vi "test - Round Trip - Array (Empty) - Cluster.vi"(8 "error in (no error)":errorcluster, 11 "TestCase in":refnum<class "Python Data Tools Tests.lvclass">) -> (0 "error out":errorcluster, 3 "TestCase out":refnum<class "Python Data Tools Tests.lvclass">)   [LabVIEW 2013, in "Python Data Tools Tests.lvclass"]
uses:
  Python Data Tools Tests.lvclass
  <vilib>/addons/_JKI Toolkits/VI Tester/TestCase.llb/TestCase.lvclass
panel:
  out "Python String":string
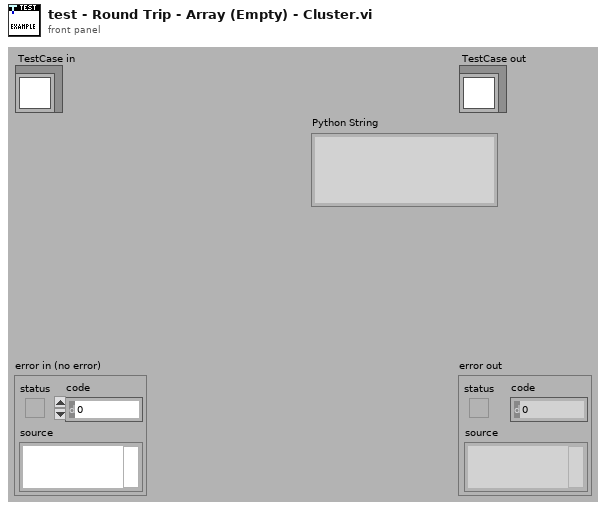
[diagram p1: front panel]
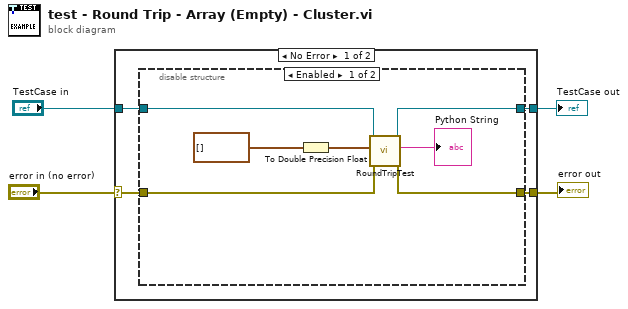
[diagram p0: block diagram]
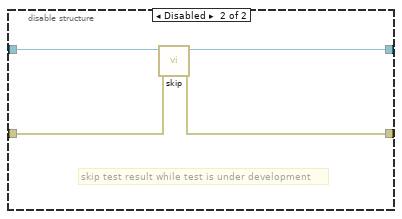
[diagram p2: hidden frame]
diagram:
  n1 = case shown="No Error" "error in (no error)" {
    selector: "error in (no error)" -> [w6 w21]
    tunnel: [w5 w21] -> w3
    tunnel: [w7 w20] -> w1
    tunnel: "TestCase in" -> [w8 w20]
    frame No Error {
      n2 = disable-structure shown="Enabled" {
        disable-tunnel: w8 -> [w15 w19]
        disable-tunnel: [w14 w16] -> w7
        disable-tunnel: w6 -> [w12 w18]
        disable-tunnel: [w13 w17] -> w5
        frame Enabled {
          n3 = To Double Precision Float(number=cluster{dbl}[] []) -> (double precision float=w11:cluster{dbl}[])
          n4 = call "RoundTripTest.vi"("error in (no error)"=w12, "Variant"=w11, "TestCase in"=w15) -> ("error out"=w13:errorcluster, "Python String"=→"Python String":string, "TestCase out"=w14:refnum<class "Python Data Tools Tests.lvclass">)  [unwired: 6 in]
        }
        frame Disabled {
          # "skip test result while test is under development"
          n5 = call <vilib>:"skip.vi"("error in (no error)"=w18, "TestCase in"=w19) -> ("error out"=w17:errorcluster, "TestCase out"=w16:refnum<class "Python Data Tools Tests.lvclass">)  [unwired: 8 in]
        }
      }
    }
    frame Error {
    }
  }
  "error out" <- w3
  "TestCase out" <- w1
